vi "Derivative (single).vi"(8 "error in (no error)":errorcluster, 9 "type":enum16{"dy/dx vs x", "dx/dy vs y"}(ring), 10 "Numeric (2)":dbl=2.0, 11 "XY-data in":cluster{"X-array":dbl[], "Y-array":dbl[]}) -> (0 "error out":errorcluster, 3 "XY-data out":cluster{"X-array":dbl[], "Y-array":dbl[]} {"Y-array" format="%.2p"; "X-array" format="%.2p"})   [LabVIEW 2016, in "xy_utilities.lvlib"]
uses:
  xy_utilities.lvlib
  <vilib>/Analysis/NI_AALPro.lvlib
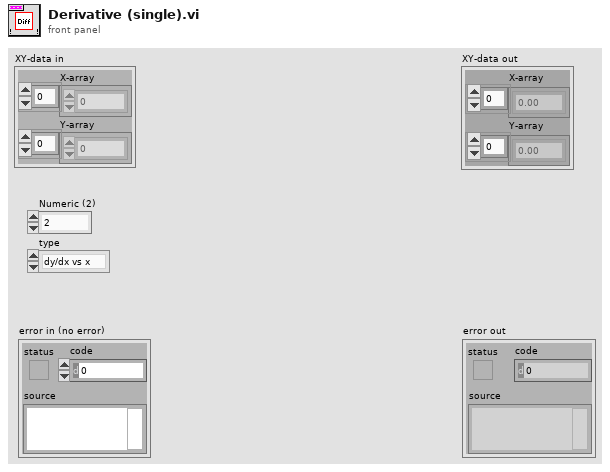
[diagram p1: front panel]
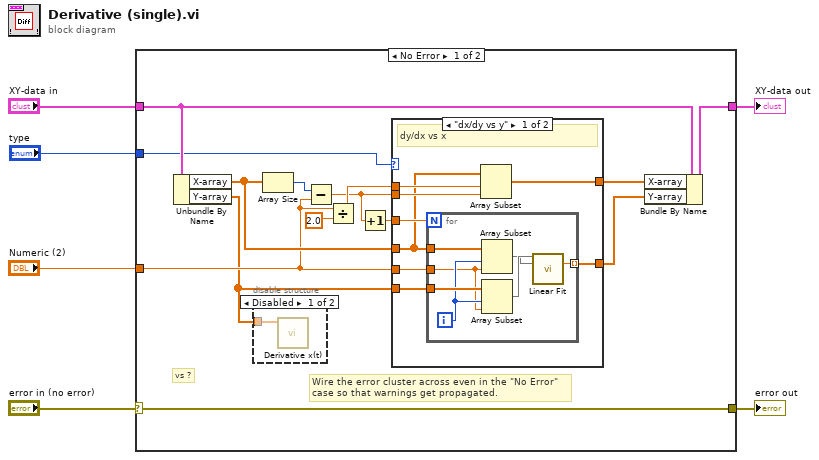
[diagram p0: block diagram]
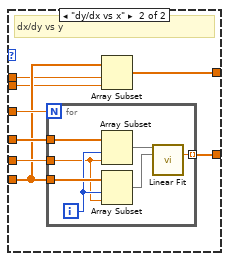
[diagram p3: hidden frame]
diagram:
  n1 = case shown="No Error" "error in (no error)" {
    selector: "error in (no error)" -> [w20 w53]
    tunnel: [w20 w53] -> w5
    tunnel: "XY-data in" -> [w19 w52]
    tunnel: [w18 w52] -> w3
    tunnel: "type" -> [w9 _]
    tunnel: "Numeric (2)" -> [w8 _]
    frame No Error {
      # "vs ?"
      # "Wire the error cluster across even in the \"No Error\"\ncase so that warnings get propagated."
      n2 = Unbundle By Name(w19) -> ("X-array"=w10:dbl[], "Y-array"=w7:dbl[])
      n3 = disable-structure shown="Disabled" {
        disable-tunnel: w7 -> [w21 _]
        frame Disabled {
          n4 = call <vilib>:"Derivative x(t).vi"("X"=w21) -> ()  [unwired: 9 in, 2 out]
        }
        frame Enabled {
        }
      }
      n5 = Array Size(array=w10) -> (size(s)=w17:i32)
      n6 = Subtract(x=w17, y=w8) -> (x-y=w13:dbl)
      n7 = Divide(x=w8, y=2.0) -> (x/y=w14:dbl)
      n8 = Increment(x=w13) -> (x+1=w16:dbl)
      n9 = case shown="\"dx/dy vs y\"" w9 {
        tunnel: w16 -> [w29 w44]
        tunnel: w8 -> [w28 w43]
        tunnel: [w27 w42] -> w12
        tunnel: w10 -> [w22 w41]
        tunnel: w7 -> [w26 w40]
        tunnel: w14 -> [w25 w38]
        tunnel: w13 -> [w24 w39]
        tunnel: [w23 w37] -> w11
        frame "dx/dy vs y" {
          # "dy/dx vs x"
          n10 = for {
            N: w29 -> [_]
            tunnel: w22 -> [w36]
            tunnel: w26 -> [w35]
            tunnel: w28 -> [w33]
            tunnel: [w32] -> w27 mode=indexing
            i -> [w34]
            n11 = Array Subset(array=w36, index=w34, length=w33) -> (w30:dbl[])
            n12 = Array Subset(array=w35, index=w34, length=w33) -> (w31:dbl[])
            n13 = call <vilib>:"Linear Fit.vi"("Y"=w31, "X"=w30) -> ("slope"=w32:dbl)  [unwired: 9 in, 4 out]
          }
          n14 = Array Subset(array=w22, index=w25, length=w24) -> (w23:dbl[])
        }
        frame "dy/dx vs x" {
          # "dx/dy vs y"
          n15 = for {
            N: w44 -> [_]
            tunnel: w41 -> [w51]
            tunnel: w40 -> [w50]
            tunnel: w43 -> [w48]
            tunnel: [w47] -> w42 mode=indexing
            i -> [w49]
            n16 = Array Subset(array=w51, index=w49, length=w48) -> (w46:dbl[])
            n17 = Array Subset(array=w50, index=w49, length=w48) -> (w45:dbl[])
            n18 = call <vilib>:"Linear Fit.vi"("Y"=w46, "X"=w45) -> ("slope"=w47:dbl)  [unwired: 9 in, 4 out]
          }
          n19 = Array Subset(array=w40, index=w38, length=w39) -> (w37:dbl[])
        }
      }
      n20 = Bundle By Name(cluster=w19, "X-array"=w11, "Y-array"=w12) -> (w18:cluster{"X-array":dbl[], "Y-array":dbl[]})
    }
    frame Error {
    }
  }
  "error out" <- w5
  "XY-data out" <- w3
